vi "Read.vi"(8 "error in (no error)":errorcluster, 11 "Path Array in":refnum<class "Path Array.lvclass">) -> (0 "error out":errorcluster, 2 "Path Array":path[](array[path]), 3 "Path Array out":refnum<class "Path Array.lvclass">)   [LabVIEW 2020, in "Data.lvlib" / "Path Array.lvclass"]
doc: "Read Path Array."
uses:
  Path Array.lvclass
  Path Array.lvclass/Path Array.ctl
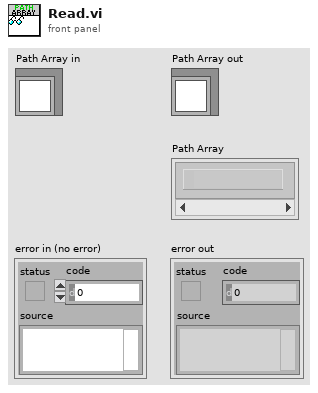
[diagram p1: front panel]
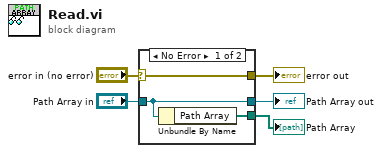
[diagram p0: block diagram]
diagram:
  n1 = case shown="No Error" "error in (no error)" {
    selector: "error in (no error)" -> [w8 w9]
    tunnel: [w8 w9] -> w4
    tunnel: [w7 w10] -> w2
    tunnel: "Path Array in" -> [w7 w10]
    tunnel: [w6 _] -> w1
    frame No Error {
      n2 = Unbundle By Name(w7) -> ("Path Array"=w6:path[])
    }
    frame Error {
    }
  }
  "error out" <- w4
  "Path Array out" <- w2
  "Path Array" <- w1
